vi "I2C readwrite.vi"(6 "Byte Count":u32, 7 "Timeout ms (1000)":i32=1000, 8 "error in (no error)":errorcluster, 9 "Bytes to Write":u8[](array[numeric]), 10 "Slave Address (7-bit)":u8, 11 "I2C in":refnum<class "I2C.lvclass">) -> (0 "error out":errorcluster, 2 "Bytes Read":u8[](array[numeric]), 3 "I2C out":refnum<class "I2C.lvclass">)   [LabVIEW 2019, in "my FPGA lib.lvlib" / "I2C.lvclass"]
uses:
  I2C.lvclass
  I2C.lvclass/I2C.ctl
  <vilib>/Utility/error.llb/Error Cluster From Error Code.vi
  <vilib>/myRIO/Common/Instrument Driver Framework/myRIO v1.0/I2C/vis/myRIO v1.0 Write I2C.vi
  <vilib>/myRIO/Common/Instrument Driver Framework/myRIO v1.0/I2C/vis/myRIO v1.0 Read I2C.vi
  <vilib>/myRIO/Instrument Drivers/Onboard IO/I2C/I2C.lvlib
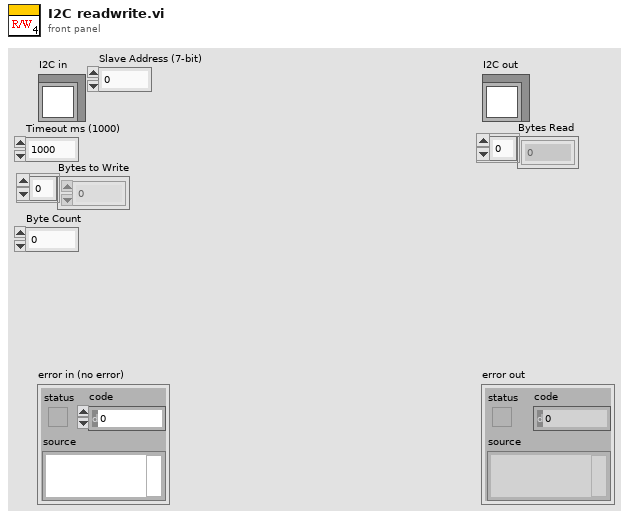
[diagram p1: front panel]
types:
  T1 = typedef "I2C.lvlib/I2C Reference.ctl" = cluster{"myRIO Reference":T2, "I2C Channels Enum":T6, "I2C Configuration":T7}
  T2 = typedef "myRIO Generic Hardware Reference.ctl" = cluster{"myRIO Model":T3, "myRIO Hardware Reference":T4}
  T3 = typedef "Hardware Version Enum.ctl" = enum16{"Unknown", "myRIO-1900", "myRIO-1950", "roboRIO", "NI ELVIS RIO CM", "ELVIS III"}
  T4 = typedef "myRIO v1.0 Reference.ctl" = cluster{"Generic FPGA Reference":T5, "Allow multiple opens":bool}
  T5 = typedef "Generic FPGA Reference.ctl" = refnum<k20>
  T6 = typedef "I2C Channels Enum.ctl" = enum16{"Not Connected", "A/I2C", "B/I2C", "I2C/I2C"}
  T7 = typedef "I2C.lvlib/I2C Configuration.ctl" = cluster{"I2C Transfer Rate":T8}
  T8 = typedef "I2C.lvlib/I2C Transfer Rate.ctl" = enum16{"Standard mode (100 kbps)", "Fast mode (400 kbps)"}
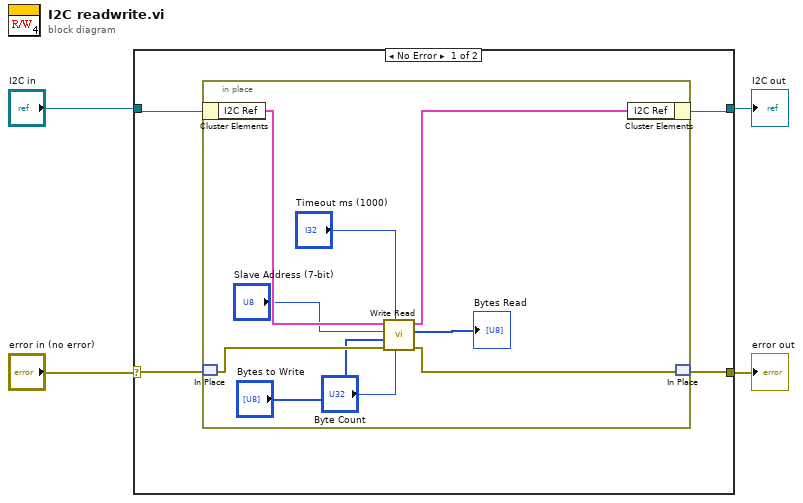
[diagram p0: block diagram]
diagram:
  n1 = case shown="No Error" "error in (no error)" {
    selector: "error in (no error)" -> [w8 w19]
    tunnel: [w7 w19] -> w3
    tunnel: [w5 w18] -> w1
    tunnel: "I2C in" -> [w6 w18]
    frame No Error {
      n2 = in-place {
        n3 = in-place-cluster #1(w6) -> ("I2C Ref"=w15:T1)
        n4 = in-place-match #2(w8) -> (w17:errorcluster)
        n5 = call <vilib>:"Write Read.vi"("Byte Count"="Byte Count", "Timeout ms (1000)"="Timeout ms (1000)", "error in (no error)"=w17, "Bytes to Write"="Bytes to Write", "Slave Address (7-bit)"="Slave Address (7-bit)", "I2C Ref In"=w15) -> ("error out"=w16:errorcluster, "Bytes Read"=→"Bytes Read":u8[], "I2C Ref Out"=w14:T1)  [unwired: 2 in]
        n6 = in-place-cluster #1("I2C Ref"=w14) -> (w5:refnum<class "I2C.lvclass">)
        n7 = in-place-match #2(w16) -> (w7:errorcluster)
      }
    }
    frame Error {
    }
  }
  "error out" <- w3
  "I2C out" <- w1
